vi "_Read_n.vi"(8 "error in (no error)":errorcluster, 11 "Postgres Connector In":refnum<class "Postgres Connector.lvclass">) -> (0 "error out":errorcluster, 2 "data out":string, 3 "Postgres Connector Out":refnum<class "Postgres Connector.lvclass">)   [LabVIEW 2020, in "Postgres Connector.lvclass"]
uses:
  Postgres Connector.lvclass
  Enum_RowDescription_State_Machine.ctl
  Cluster_Reader_Infos.ctl
  Postgres Connector.lvclass/Postgres Connector.ctl
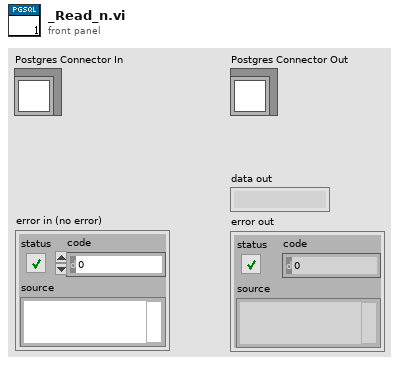
[diagram p1: front panel]
types:
  T1 = typedef "Postgres Connector.lvclass/Cluster_Reader_Infos.ctl" = cluster{"Byte Length":i32}
  T2 = typedef "Postgres Connector.lvclass/Enum_RowDescription_State_Machine.ctl" = enum16{"Check For Error", "Wait For T", "Wait For D", "Wait For Z", "C Byte Length", "Z Byte Length", "n Byte Length", "Byte Length", "Get Infos", "Check For End", "Flush", "Quit"}
  T3 = enum16{"Standard", "Buffered", "CRLF", "Immediate"}
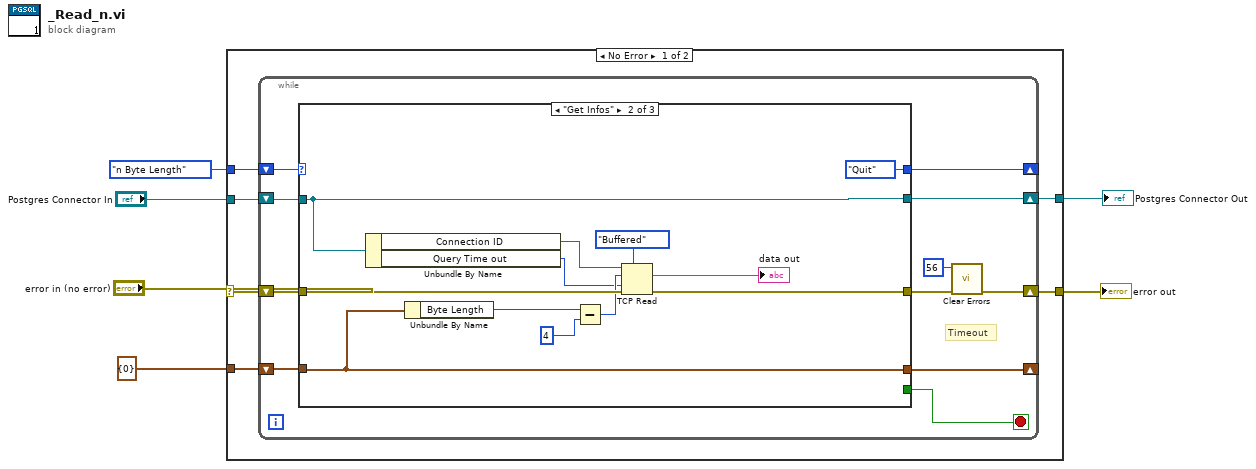
[diagram p0: block diagram]
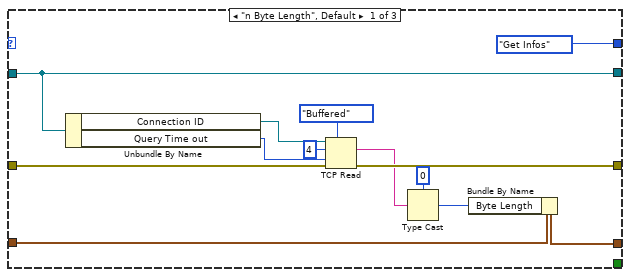
[diagram p2: hidden frame]
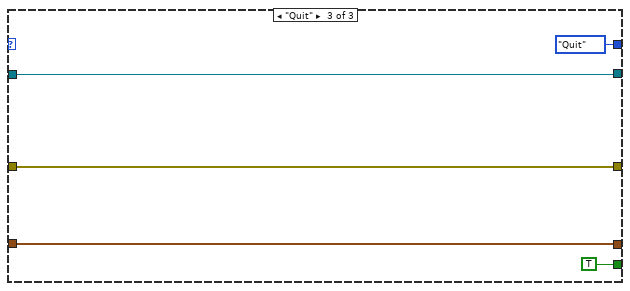
[diagram p3: hidden frame]
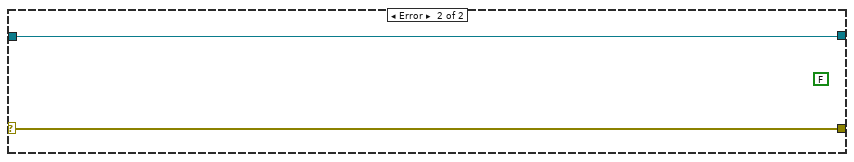
[diagram p4: hidden frame]
diagram:
  n1 = case shown="No Error" "error in (no error)" {
    selector: "error in (no error)" -> [w11 w55]
    tunnel: "Postgres Connector In" -> [w12 w54]
    tunnel: Enum_RowDescription_State_Machine."n Byte Length" -> [w10 _]
    tunnel: [w9 w55] -> w3
    tunnel: T1 {"Byte Length"=0} ("Reader_Infos") -> [w8 _]
    tunnel: [w7 w54] -> w1
    frame No Error {
      n2 = while {
        shift-right: [w19] -> w9
        shift-left: w11 -> [w22]
        shift-right: [w17] -> _
        shift-left: w10 -> [w21]
        shift-right: [w15] -> _
        shift-left: w8 -> [w16]
        shift-right: [w13] -> w7
        shift-left: w12 -> [w23]
        stop <- w14 stop-if-true
        # "Timeout"
        n3 = case shown="\"Get Infos\"" w21 {
          tunnel: w23 -> [w32 w38 w49]
          tunnel: w22 -> [w33 w46 w52]
          tunnel: [w31 w45 w52] -> w20
          tunnel: [Enum_RowDescription_State_Machine."Get Infos" Enum_RowDescription_State_Machine."Quit" Enum_RowDescription_State_Machine."Quit"] -> w17
          tunnel: w16 -> [w30 w43 w53]
          tunnel: [w29 w43 w53] -> w15
          tunnel: [_ _ TRUE] -> w14
          tunnel: [w32 w38 w49] -> w13
          frame "n Byte Length", Default {
            n4 = Unbundle By Name(w32) -> ("Connection ID"=w35:refnum<k5>, "Query Time out"=w24:i32)
            n5 = TCP Read(connection ID=w35, bytes to read=4, error in (no error)=w33, 7:T3."Buffered" ("mode (standard)"), 9:w24) -> (data out=w25:string, error out=w31:errorcluster)  [unwired: 1 out]
            n6 = Type Cast(type=0, x=w25) -> (*(type *) &x=w26:i32)
            n7 = Bundle By Name(cluster=w30, "Byte Length"=w26) -> (w29:T1)
          }
          frame "Get Infos" {
            n8 = Unbundle By Name(w38) -> ("Connection ID"=w47:refnum<k5>, "Query Time out"=w39:i32)
            n9 = Unbundle By Name(w43) -> ("Byte Length"=w42:i32)
            n10 = Subtract(x=w42, y=4 ("bytes to read")) -> (x-y=w41:i32)
            n11 = TCP Read(connection ID=w47, bytes to read=w41, error in (no error)=w46, 7:T3."Buffered" ("mode (standard)"), 9:w39) -> (data out=→"data out":string, error out=w45:errorcluster)  [unwired: 1 out]
          }
          frame "Quit" {
          }
        }
        n12 = call <vilib>:"Clear Errors.vi"("error in (no error)"=w20, "specific error code to clear (0: all)"=56) -> ("error out"=w19:errorcluster)  [unwired: 4 in, 1 out]
      }
    }
    frame Error {
      (unwired) FALSE
    }
  }
  "error out" <- w3
  "Postgres Connector Out" <- w1
